vi "Parse TXT Configuration File_Parse DMA Channels.vi"(8 "error in (no error)":errorcluster, 10 "DMA Blocks":T2[](array[typedef]), 11 "Array in":string[][](array[string])) -> (0 "error out":errorcluster, 3 "DMAs":T1[](array[typedef]))   [LabVIEW 2020, in "RefMem DMA System Explorer.lvlib"]
uses:
  RefMem DMA System Explorer.lvlib
  controls/Typedef_DMA Block Settings.ctl
  controls/Typedef_Channel Settings.ctl
  controls/Typedef_DMA Instance.ctl
  controls/Data Channel Type.ctl
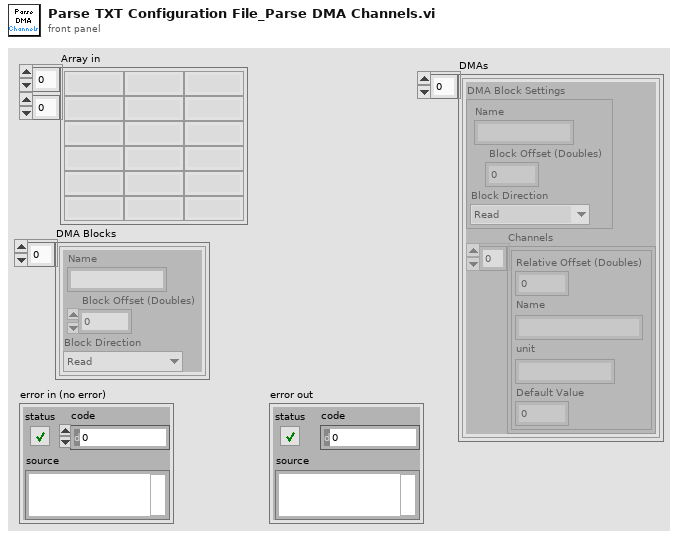
[diagram p1: front panel]
types:
  T1 = typedef "RefMem DMA System Explorer.lvlib/Typedef_DMA Instance.ctl" = cluster{"DMA Block Settings":T2, "Channels":T4[]}
  T2 = typedef "RefMem DMA System Explorer.lvlib/Typedef_DMA Block Settings.ctl" = cluster{"Name":string, " Block Offset (Doubles)":u32, "Block Direction":T3}
  T3 = typedef "RefMem DMA System Explorer.lvlib/Data Channel Type.ctl" = enum16{"Read", "Write"}
  T4 = typedef "RefMem DMA System Explorer.lvlib/Typedef_Channel Settings.ctl" = cluster{"Relative Offset (Doubles)":u32, "Name":string, "unit":string, "Default Value":dbl}
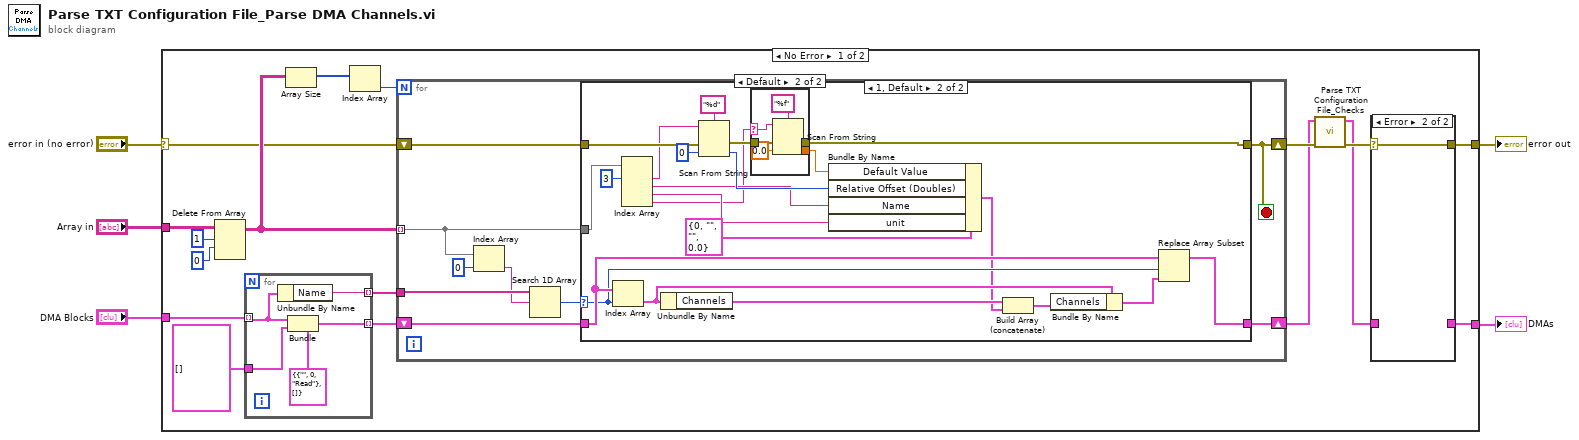
[diagram p0: block diagram]
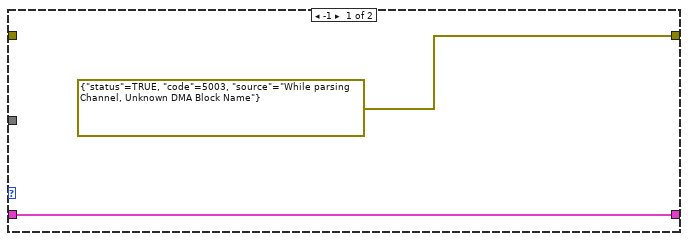
[diagram p2: hidden frame]
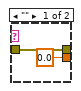
[diagram p3: hidden frame]
diagram:
  n1 = case shown="No Error" "error in (no error)" {
    selector: "error in (no error)" -> [w10 w72]
    tunnel: "Array in" -> [w20 _]
    tunnel: [w19 w72] -> w4
    tunnel: "DMA Blocks" -> [w18 _]
    tunnel: [w11 _] -> w1
    frame No Error {
      n2 = Delete From Array(array=w20, length=1, index (row)=0) -> (array with subset deleted=w14:string[][])  [unwired: 1 in, 1 out]
      n3 = for {
        tunnel: w18 -> [w24] mode=indexing
        tunnel: T4[] [] -> [w27]
        tunnel: [w25] -> w16 mode=indexing
        tunnel: [w23] -> w15 mode=indexing
        n4 = Unbundle By Name(w24) -> ("Name"=w23:string)
        n5 = Bundle(cluster=T1 {"DMA Block Settings"={"Name"="", " Block Offset (Doubles)"=0, "Block Direction"=enum."Read"}, "Channels"=[]} ("DMA"), "DMA Block Settings"=w24, "Channels"=w27) -> (w25:T1)
      }
      n6 = Array Size(array=w14) -> (size(s)=w13:i32[])
      n7 = Index Array(array=w13) -> (element=w12:i32)  [unwired: 1 in]
      n8 = for {
        N: w12 -> [_]
        tunnel: w14 -> [w28] mode=indexing
        shift-right: [w29] -> w7
        shift-left: w16 -> [w30]
        tunnel: w15 -> [w35]
        shift-right: [w31] -> w9
        shift-left: w10 -> [w32]
        stop <- w31 stop-if-true
        n9 = Index Array(array=w28, index=0) -> (element=w34:string)
        n10 = Search 1D Array(1D array=w35, element=w34) -> (index of element=w33:i32)  [unwired: 1 in]
        n11 = case shown="1, Default" w33 {
          selector: w33 -> [_ w56]
          tunnel: w32 -> [_ w51]
          tunnel: [errorcluster {"status"=TRUE, "code"=5003, "source"="While parsing Channel, Unknown DMA Block Name"} ("error IO") w40] -> w31
          tunnel: w30 -> [w37 w57]
          tunnel: [w37 w54] -> w29
          tunnel: w28 -> [_ w53]
          frame -1 {
          }
          frame 1, Default {
            n12 = Index Array(array=w57, index=w56) -> (element=w59:T1)
            n13 = Index Array(array=w53, index #1=3 ("index")) -> (element #1=w49:string, element #2=w42:string, element #3=w41:string, element #4=w39:string)  [unwired: 3 in]
            n14 = Unbundle By Name(w59) -> ("Channels"=w60:T4[])
            n15 = Scan From String(format string="%d", input string=w49, error in=w51, default 1=u32 0) -> (error out=w45:errorcluster, output 1=w43:u32)  [unwired: 1 in, 2 out]
            n16 = case shown="Default" w39 {
              selector: w39 -> [_ w63]
              tunnel: w45 -> [w61 w68]
              tunnel: [0.0 w65] -> w44
              tunnel: [w61 w64] -> w40
              frame "" {
              }
              frame Default {
                n17 = Scan From String(format string="%f", input string=w63, error in=w68, default 1=0.0) -> (error out=w64:errorcluster, output 1=w65:dbl)  [unwired: 1 in, 2 out]
              }
            }
            n18 = Bundle By Name(cluster=T4 {"Relative Offset (Doubles)"=0, "Name"="", "unit"="", "Default Value"=0.0} ("Channel"), "Default Value"=w44, "Relative Offset (Doubles)"=w43, "Name"=w42, "unit"=w41) -> (w46:T4)
            n19 = Build Array (concatenate)(w60, w46) -> (w58:T4[])
            n20 = Bundle By Name(cluster=w59, "Channels"=w58) -> (w55:T1)
            n21 = Replace Array Subset(array=w57, new element=w55, index=w56) -> (w54:T1[])
          }
        }
      }
      n22 = call "Parse TXT Configuration File_Checks.vi"("error in (no error)"=w9, "DMAs In"=w7) -> ("error out"=w8:errorcluster, "DMAs Out"=w6:T1[])  [unwired: 8 in]
      n23 = case shown="Error" w8 {
        selector: w8 -> [w70 w71]
        tunnel: [w70 w71] -> w19
        tunnel: w6 -> [w69 _]
        tunnel: [w69 _] -> w11
        frame No Error {
        }
        frame Error {
        }
      }
    }
    frame Error {
    }
  }
  "error out" <- w4
  "DMAs" <- w1
